vi "Find Log File by Name.vi"(8 "error in":errorcluster, 10 "log file name":string="Log File", 11 "embedded data logger in":T1=18446744073709551615 format="%.0x") -> (0 "error out":errorcluster, 2 "log file":T1 format="%.0x", 3 "embedded data logger out":T1 format="%.0x")   [LabVIEW 2027, in "Embedded Data Logger Scripting.lvlib"]
uses:
  Embedded Data Logger Scripting.lvlib
  <vilib>/NI VeriStand/Custom Device API/Custom Device Item Ref.ctl
  <vilib>/NI VeriStand/Custom Device API/Custom Device API.lvlib
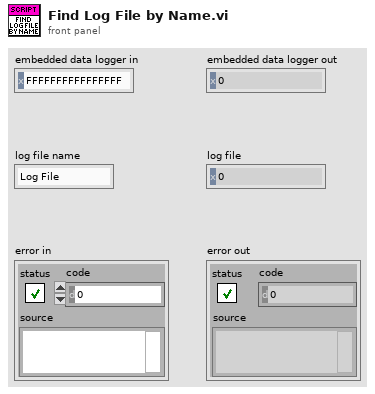
[diagram p1: front panel]
types:
  T1 = typedef "Custom Device API.lvlib/Custom Device Item Ref.ctl" = u64
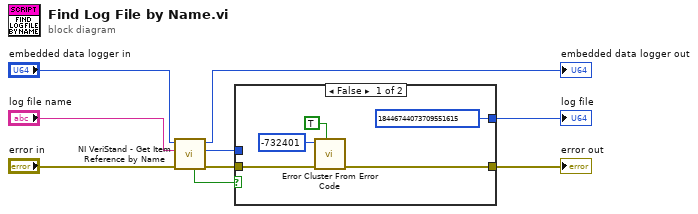
[diagram p0: block diagram]
diagram:
  n1 = call <vilib>:"NI VeriStand - Get Item Reference by Name.vi"("error in (no error)"="error in", "Item Name"="log file name", "Parent Ref in"="embedded data logger in") -> ("error out"=w4:errorcluster, "Item Ref"=w1:T1, "Parent Ref out"=→"embedded data logger out":T1, "Found"=w6:bool)  [unwired: 5 in]
  n2 = case shown="False" w6 {
    tunnel: [w14 w16] -> w5
    tunnel: w4 -> [w13 w16]
    tunnel: [T1 18446744073709551615 ("Item Ref") w15] -> w2
    tunnel: w1 -> [_ w15]
    frame False {
      n3 = call <vilib>:"Error Cluster From Error Code.vi"("show call chain? (False)"=TRUE, "error in (no error)"=w13, "error code (0)"=-732401) -> ("error out"=w14:errorcluster)  [unwired: 6 in]
    }
    frame True {
    }
  }
  "log file" <- w2
  "error out" <- w5
